vi "Global - Test.vi"() -> ()   [LabVIEW 2019]
panel:
  out "Test":T1(array[cluster])
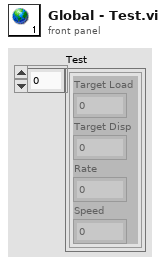
[diagram p1: front panel]
types:
  T1 = cluster{"Target Load":sgl, "Target Disp":sgl, "Rate":sgl, "Speed":sgl}[]
diagram:
